vi "ManualLauncher.vi"() -> ()   [LabVIEW 2012]
uses:
  LauncherPresets.ctl
  Robot Global Data.vi
panel:
  in  "LauncherPresets":T1
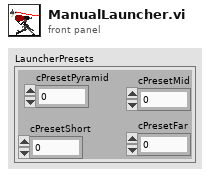
[diagram p1: front panel]
types:
  T1 = typedef "LauncherPresets.ctl" = cluster{"cPresetPyramid":dbl, "cPresetShort":dbl, "cPresetMid":dbl, "cPresetFar":dbl}
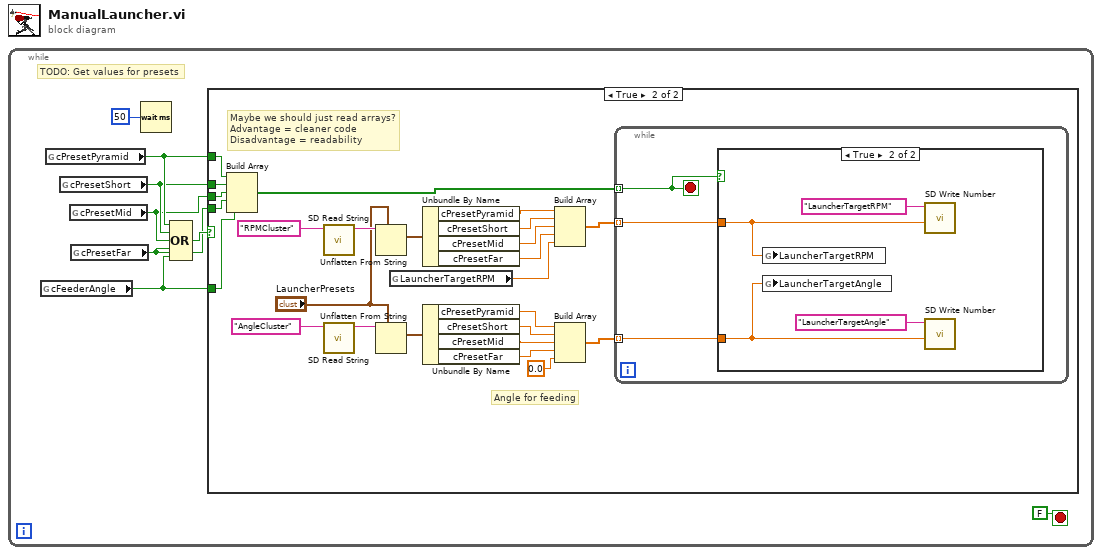
[diagram p0: block diagram]
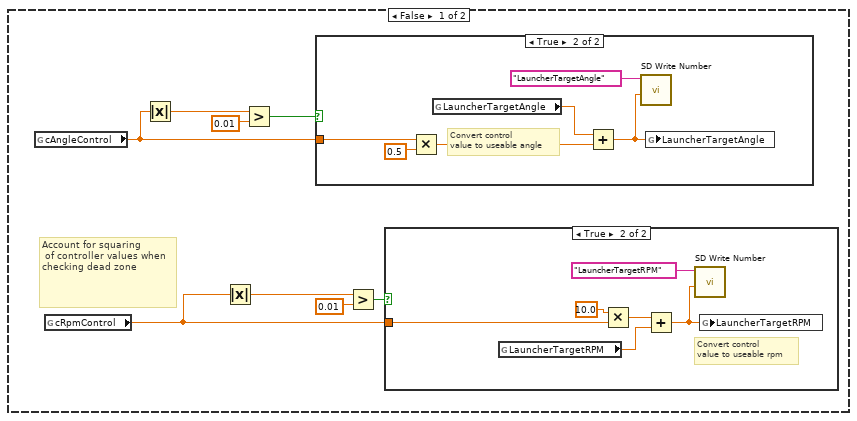
[diagram p2: hidden frame]
diagram:
  n1 = while {
    stop <- FALSE stop-if-true
    # "TODO: Get values for presets"
    n2 = global read "Robot Global Data.vi" "cFeederAngle"() -> (w1:bool)
    n3 = global read "Robot Global Data.vi" "cPresetPyramid"() -> (w6:bool)
    n4 = global read "Robot Global Data.vi" "cPresetShort"() -> (w5:bool)
    n5 = global read "Robot Global Data.vi" "cPresetMid"() -> (w4:bool)
    n6 = global read "Robot Global Data.vi" "cPresetFar"() -> (w3:bool)
    n7 = Wait (ms)(milliseconds to wait=u32 50) -> ()  [unwired: 1 out]
    n8 = Compound Arithmetic op=OR(w6, w5, w4, w3, w1) -> (w7:bool)
    n9 = case shown="True" w7 {
      tunnel: w6 -> [_ w53]
      tunnel: w5 -> [_ w52]
      tunnel: w4 -> [_ w51]
      tunnel: w3 -> [_ w50]
      tunnel: w1 -> [_ w31]
      frame False {
        # "Account for squaring\n of controller values when checking dead zone"
        n10 = global read "Robot Global Data.vi" "cAngleControl"() -> (w12:dbl)
        n11 = global read "Robot Global Data.vi" "cRpmControl"() -> (w14:dbl)
        n12 = Absolute Value(x=w12) -> (abs(x)=w13:dbl)
        n13 = Absolute Value(x=w14) -> (abs(x)=w15:dbl)
        n14 = Greater?(x=w13, y=0.01) -> (0:w11:bool)
        n15 = case shown="True" w11 {
          tunnel: w12 -> [_ w22]
          frame False {
          }
          frame True {
            # "Convert control\nvalue to useable angle"
            n16 = Multiply(x=w22, y=0.5) -> (x*y=w19:dbl)
            n17 = global read "Robot Global Data.vi" "LauncherTargetAngle"() -> (w20:dbl)
            n18 = Add(x=w20, y=w19) -> (x+y=w17:dbl)
            n19 = call <vilib>:"SD Write Number.vi"("Numeric"=w17, "Name"="LauncherTargetAngle") -> ()  [unwired: 8 in, 2 out]
            n20 = global write "Robot Global Data.vi" "LauncherTargetAngle"(w17) -> ()
          }
        }
        n21 = Greater?(x=w15, y=0.01) -> (0:w10:bool)
        n22 = case shown="True" w10 {
          tunnel: w14 -> [_ w27]
          frame False {
          }
          frame True {
            # "Convert control\nvalue to useable rpm"
            n23 = global read "Robot Global Data.vi" "LauncherTargetRPM"() -> (w26:dbl)
            n24 = Multiply(x=10.0, y=w27) -> (x*y=w25:dbl)
            n25 = Add(x=w25, y=w26) -> (x+y=w23:dbl)
            n26 = call <vilib>:"SD Write Number.vi"("Numeric"=w23, "Name"="LauncherTargetRPM") -> ()  [unwired: 8 in, 2 out]
            n27 = global write "Robot Global Data.vi" "LauncherTargetRPM"(w23) -> ()
          }
        }
      }
      frame True {
        # "Angle for feeding"
        # "Maybe we should just read arrays?\nAdvantage = cleaner code\nDisadvantage = readability"
        n28 = Build Array(w53, w52, w51, w50, w31) -> (w49:bool[])
        n29 = call <vilib>:"SD Read String.vi"("Name"="RPMCluster") -> ("String"=w39:string)  [unwired: 8 in, 2 out]
        n30 = call <vilib>:"SD Read String.vi"("Name"="AngleCluster") -> ("String"=w47:string)  [unwired: 8 in, 2 out]
        n31 = Unflatten From String(type="LauncherPresets", binary string=w39) -> (value=w37:T1)  [unwired: 3 in, 2 out]
        n32 = Unflatten From String(type="LauncherPresets", binary string=w47) -> (value=w46:T1)  [unwired: 3 in, 2 out]
        n33 = global read "Robot Global Data.vi" "LauncherTargetRPM"() -> (w30:dbl)
        n34 = Unbundle By Name(w37) -> ("cPresetPyramid"=w36:dbl, "cPresetShort"=w35:dbl, "cPresetMid"=w34:dbl, "cPresetFar"=w33:dbl)
        n35 = Unbundle By Name(w46) -> ("cPresetPyramid"=w45:dbl, "cPresetShort"=w44:dbl, "cPresetMid"=w43:dbl, "cPresetFar"=w42:dbl)
        n36 = Build Array(w36, w35, w34, w33, w30) -> (w32:dbl[])
        n37 = Build Array(w45, w44, w43, w42, 0.0 ("element")) -> (w41:dbl[])
        n38 = while {
          tunnel: w49 -> [w56] mode=indexing
          tunnel: w41 -> [w55] mode=indexing
          tunnel: w32 -> [w54] mode=indexing
          stop <- w56 stop-if-true
          n39 = case shown="True" w56 {
            tunnel: w55 -> [_ w57]
            tunnel: w54 -> [_ w59]
            frame False {
            }
            frame True {
              n40 = global write "Robot Global Data.vi" "LauncherTargetRPM"(w59) -> ()
              n41 = global write "Robot Global Data.vi" "LauncherTargetAngle"(w57) -> ()
              n42 = call <vilib>:"SD Write Number.vi"("Numeric"=w59, "Name"="LauncherTargetRPM") -> ()  [unwired: 8 in, 2 out]
              n43 = call <vilib>:"SD Write Number.vi"("Numeric"=w57, "Name"="LauncherTargetAngle") -> ()  [unwired: 8 in, 2 out]
            }
          }
        }
      }
    }
  }
